vi "process.vi"(8 "error in":errorcluster, 9 "result allocation":T2, 10 "parameters":T2, 11 "Watchdog runtime in":refnum<class "Watchdog runtime.lvclass">) -> (0 "error out":errorcluster, 1 "results":T2, 2 "parameter allocation":T2, 3 "Watchdog runtime out":refnum<class "Watchdog runtime.lvclass">)   [LabVIEW 2013, in "Watchdog runtime.lvclass"]
doc: "Provides an interface for information processing by a module at runtime. While this interface performs no operations, a child should provide an override which may process data in any manner necessary."
uses:
  Watchdog runtime.lvclass
  <vilib>/NI/Tag Bus/table/data table.ctl
  <vilib>/RTwatchdog.llb/Watchdog status enum.ctl
  Watchdog runtime.lvclass/Watchdog runtime.ctl
  <vilib>/NI/Tag Bus/table/data table.lvlib
panel:
  out "watchdog status":T1
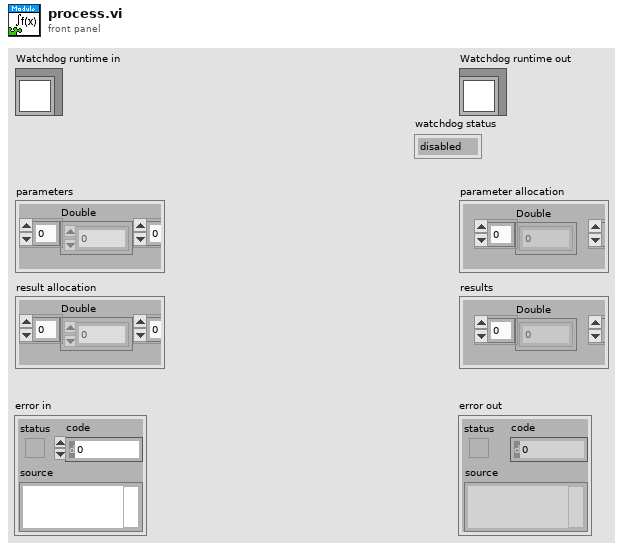
[diagram p1: front panel]
types:
  T1 = typedef "Watchdog status enum.ctl" = enum16{"disabled", "expired", "running"}
  T2 = typedef "tag bus.lvlib/data table.lvlib/data table.ctl" = cluster{"Double":dbl[], "Single":sgl[], "I64":i64[], "I32":i32[], "I16":i16[], "I8":i8[], "U64":u64[], "U32":u32[], "U16":u16[], "U8":u8[], "Boolean":bool[], "String":string[], "Array of Double":cluster{"DBL Array":dbl[]}[], "Array of Single":cluster{"SGL Array":sgl[]}[], "Array of I64":cluster{"I64 Array":i64[]}[], "Array of I32":cluster{"I32 Array":i32[]}[], "Array of I16":cluster{"I16 Array":i16[]}[], "Array of I8":cluster{"I8 Array":i8[]}[], "Array of U64":cluster{"U64 Array":u64[]}[], "Array of U32":cluster{"U32 Array":u32[]}[], "Array of U16":cluster{"U16 Array":u16[]}[], "Array of U8":cluster{"U8 Array":u8[]}[], "Array of Boolean":cluster{"Boolean Array":bool[]}[], "Array of String":cluster{"String Array":string[]}[]}
  T3 = typedef "Watchdog configuration.lvclass/parameter data indices.ctl" = cluster{"placeholder":i32}
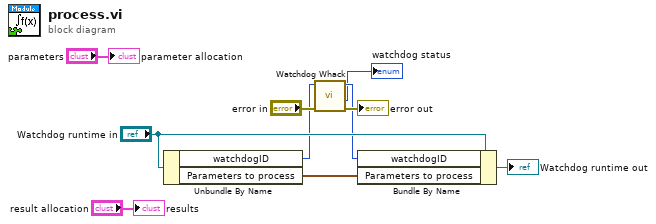
[diagram p0: block diagram]
diagram:
  n1 = Unbundle By Name("Watchdog runtime in") -> ("watchdogID"=w6:u32, "Parameters to process"=w4:T3)
  n2 = call <vilib>:"Watchdog Whack.vi"("error in (no error)"="error in", "watchdogID in"=w6) -> ("error out"=→"error out":errorcluster, "watchdog status"=→"watchdog status":T1, "watchdogID out"=w3:u32)  [unwired: 3 in]
  n3 = Bundle By Name(cluster="Watchdog runtime in", "watchdogID"=w3, "Parameters to process"=w4) -> (→"Watchdog runtime out":refnum<class "Watchdog runtime.lvclass">)
  "results" <- "result allocation"
  "parameter allocation" <- "parameters"
